vi "Read Write Sample Code.vi"(8 "error in (no error)":errorcluster) -> (0 "error out":errorcluster)   [LabVIEW 2020]
uses:
  cf616b22-67e3-4c3f-9906-26a713c7887b.vi
  24f44c96-8ad6-4aa5-8acd-65b2b5cb4848.vi
panel:
  in  "讀取目標字數":i32
  in  "stop":bool
  in  "Write":bool
  in  "VISA resource name":refnum<visa-resource-name>
  out "read buffer":string
  in  "write buffer":string
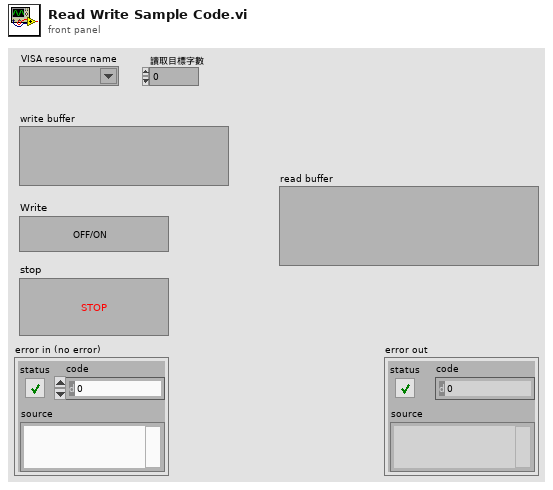
[diagram p1: front panel]
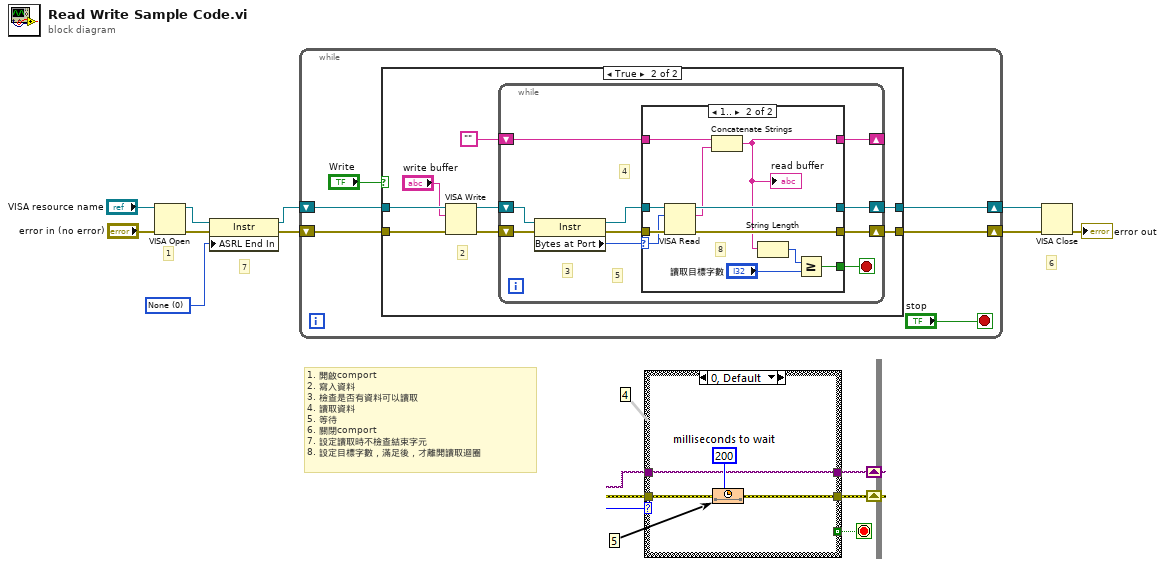
[diagram p0: block diagram]
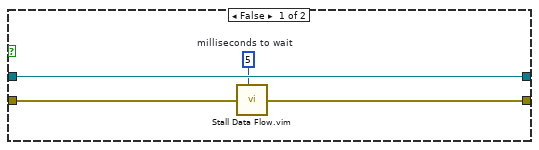
[diagram p2: hidden frame]
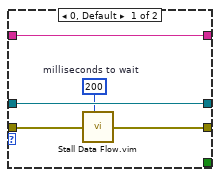
[diagram p3: hidden frame]
diagram:
  w1 = u16 0 items=["None", "Last Bit", "TermChar"] ("Serial Settings:End Mode for Reads")
  # "7"
  # "1. 開啟comport\n2. 寫入資料\n3. 檢查是否有資料可以讀取\n4. 讀取資料\n5. 等待\n6. 關閉comport\n7. 設定讀取時不檢查結束字元\n8. 設定目標字數，滿足後，才離開讀取迴圈"
  # "6"
  # "1"
  n1 = VISA Open(error in (no error)="error in (no error)", VISA resource name="VISA resource name") -> (VISA resource name=w3:refnum<visa-resource-name>, error out=w10:errorcluster)  [unwired: 3 in]
  n2 = property class="Instr"(reference=w3, error in=w10, "ASRL End In"=w1) -> (reference out=w2:refnum<visa-resource-name>, error out=w4:errorcluster)
  n3 = while {
    shift-right: [w13] -> w9
    shift-left: w2 -> [w16]
    shift-right: [w14] -> w8
    shift-left: w4 -> [w15]
    stop <- "stop" stop-if-true
    n4 = case shown="True" "Write" {
      tunnel: w16 -> [w20 w28]
      tunnel: w15 -> [w19 w27]
      tunnel: [w18 w23] -> w14
      tunnel: [w20 w22] -> w13
      frame False {
        w17 = u32 5  # milliseconds to wait
        n5 = call "Stall Data Flow.vim"("value in"=w19, "milliseconds to wait"=w17) -> ("value out"=w18:errorcluster)  [unwired: 1 out]
      }
      frame True {
        # "2"
        n6 = VISA Write(VISA resource name=w28, write buffer="write buffer", error in (no error)=w27) -> (VISA resource name out=w25:refnum<visa-resource-name>, error out=w24:errorcluster)  [unwired: 1 out]
        n7 = while {
          shift-right: [w32] -> w22
          shift-left: w25 -> [w38]
          shift-right: [w34] -> w23
          shift-left: w24 -> [w37]
          shift-right: [w30] -> _
          shift-left: "" -> [w29]
          stop <- w31 stop-if-true
          # "5"
          # "4"
          # "3"
          n8 = property class="Instr"(reference=w38, error in=w37) -> (reference out=w33:refnum<visa-resource-name>, error out=w35:errorcluster, "Bytes at Port"=w36:u32)
          n9 = case shown="1.." w36 {
            selector: w36 -> [_ w50]
            tunnel: w35 -> [w43 w54]
            tunnel: [w41 w53] -> w34
            tunnel: w33 -> [w42 w52]
            tunnel: [w42 w51] -> w32
            tunnel: [_ w46] -> w31
            tunnel: [w39 w48] -> w30
            tunnel: w29 -> [w39 w49]
            frame 0, Default {
              w40 = u32 200  # milliseconds to wait
              n10 = call "Stall Data Flow.vim"("value in"=w43, "milliseconds to wait"=w40) -> ("value out"=w41:errorcluster)  [unwired: 1 out]
            }
            frame 1.. {
              # "8"
              n11 = VISA Read(VISA resource name=w52, byte count=w50, error in (no error)=w54) -> (VISA resource name out=w51:refnum<visa-resource-name>, read buffer=w44:string, error out=w53:errorcluster)  [unwired: 1 out]
              n12 = Concatenate Strings(w49, w44) -> (w48:string)
              "read buffer" <- w48
              n13 = String Length(string=w48) -> (length=w47:i32)
              n14 = Greater Or Equal?(x=w47, y="讀取目標字數") -> (x >= y?=w46:bool)
            }
          }
        }
      }
    }
  }
  n15 = VISA Close(VISA resource name=w9, error in (no error)=w8) -> (error out=→"error out":errorcluster)
